vi "Yokogawa - measurement test.vi"() -> ()   [LabVIEW 2013]
uses:
  <instrlib>/Yokogawa PZ4000/Yokogawa PZ4000.lvlib
  electrical2.ctl
panel:
  in  "Module to save":i32=1 min=1 max=4 step=1
  in  "error in (no error)":errorcluster
  out "Electrical Data 3":T1={"Time Stamp"=timestamp(0 s since 1904-01-01), "Temperature (C)"=0.0, "Electrical Data"=[["   NaN", "   NaN", "   NaN", "   NaN"], ["   NaN", "   NaN", "   NaN", "   NaN"], ["   NaN", "   NaN", "   NaN", "   NaN"], ["   NaN", "   NaN", "   NaN", "   NaN"], ["   NaN", "   NaN", "   NaN", "   NaN"], ["   NaN", "   NaN", "   NaN", "   NaN"], ["   NaN", "   NaN", "   NaN", "   NaN"], ["   NaN", "   NaN", "   NaN", "   NaN"], ["   NaN", "   NaN", "   NaN", "   NaN"], ["   NaN", "   NaN", "   NaN", "   NaN"]], "Waveform Graph"=[]}
  in  "Mode (0: Normal)":u16(ring) items=["Normal", "Harmonics"]
  in  "Observation Time":u16(ring)=10 items=["1ksec", "400sec", "200sec", "100sec", "40sec", "20sec", "10sec", "4sec", "2sec", "1sec", "400msec", "200msec", "100msec", "40msec", "20msec", "10msec", "4msec", "2msec", "1msec", "400usec", "200usec", "100usec", "40usec", "20usec", "10usec"]
  in  "Modules on/off":T2
  in  "VISA resource name":refnum<visa-resource-name>
  in  "Current":T3={"A Range (2)"=7, "A Terminal (0: 5A)"=0, "Element (0: ALL)"=0} {"Element (0: ALL)" items=["All", "Element 1", "Element 2", "Element 3", "Element 4"]; "A Terminal (0: 5A)" items=["5A", "20A", "Sensor"]; "A Range (2)" items=["AUTO", "0.1", "0.2", "0.4", "1", "2", "4", "10", "20", "40", "100"]}
  in  "Voltage":T4={"Element (0: All)"=0, "V Range (200)"=4} {"V Range (200)" items=["AUTO", "30", "60", "120", "200", "300", "600", "1200", "2000"]; "Element (0: All)" items=["All", "Element 1", "Element 2", "Element 3", "Element 4"]}
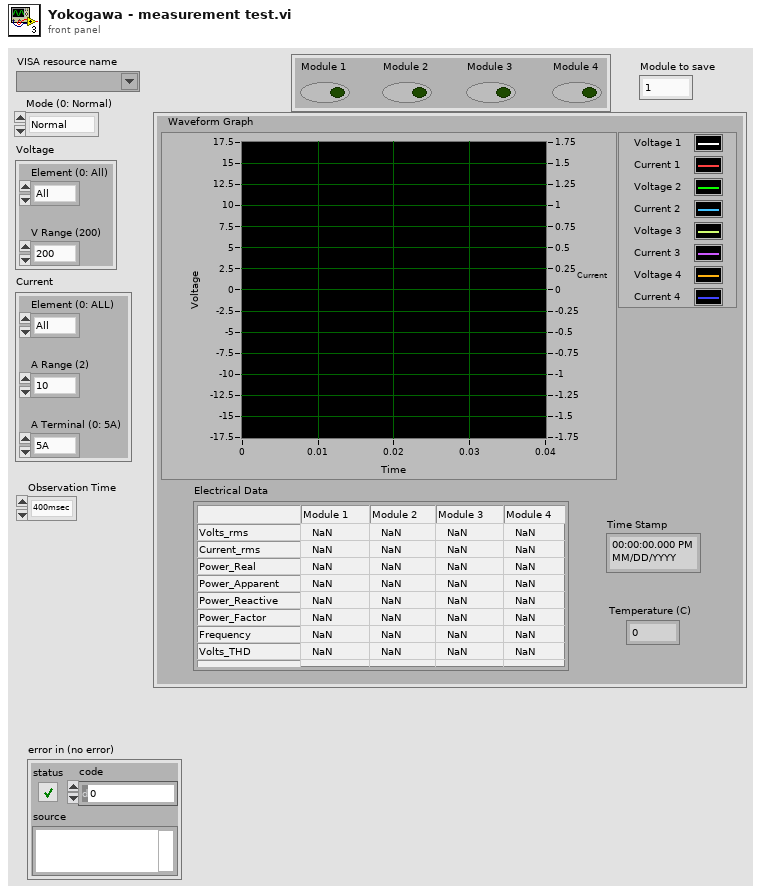
[diagram p1: front panel]
types:
  T1 = typedef "electrical2.ctl" = cluster{"Time Stamp":timestamp, "Temperature (C)":dbl, "Electrical Data":string[][], "Waveform Graph":waveform(dbl)[]}
  T2 = cluster{"Module 1":bool, "Module 2":bool, "Module 3":bool, "Module 4":bool}
  T3 = cluster{"A Range (2)":u16, "A Terminal (0: 5A)":u16, "Element (0: ALL)":u16}
  T4 = cluster{"Element (0: All)":u16, "V Range (200)":u16}
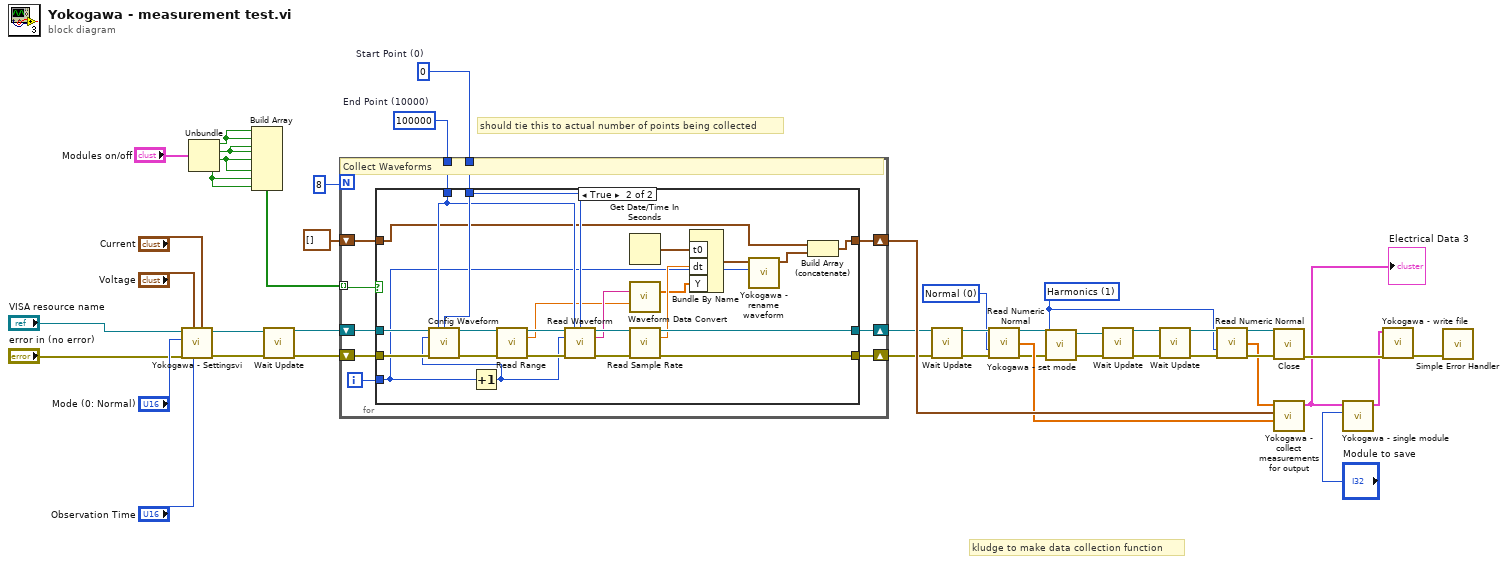
[diagram p0: block diagram]
diagram:
  w38 = u32 100000  # End Point (10000)
  w39 = u32 0  # Start Point (0)
  w8 = u16 1 items=["Normal", "Harmonics"] ("Mode (0: Normal)  2")
  w15 = u16 0 items=["Normal", "Harmonics"] ("Mode (0: Normal)")
  # "should tie this to actual number of points being collected"
  # "kludge to make data collection function"
  n1 = call "Yokogawa - Settingsvi.vi"(5:"Current", 6:"Observation Time", 7:"Voltage", "error in (no error)"="error in (no error)", 10:"Mode (0: Normal)", "Hardware Configuration"="VISA resource name") -> ("error out 2"=w20:errorcluster, "VISA resource name out"=w21:refnum<visa-resource-name>)  [unwired: 4 in]
  n2 = Unbundle("Modules on/off") -> ("Module 1"=w32:bool, "Module 2"=w31:bool, "Module 3"=w30:bool, "Module 4"=w29:bool)
  n3 = Build Array(w32, w32, w31, w31, w30, w30, w29, w29) -> (w34:bool[])
  n4 = call <instrlib>:"Wait Update.vi"("VISA resource name"=w21, "error in (no error)"=w20) -> ("VISA resource name out"=w37:refnum<visa-resource-name>, "error out"=w36:errorcluster)  [unwired: 12 in]
  n5 = for {
    N: 8 -> [_]
    tunnel: w39 -> [w54]
    tunnel: w38 -> [w53]
    shift-right: [w50] -> w24
    shift-left: w37 -> [w52]
    shift-right: [w49] -> w23
    shift-left: w36 -> [w51]
    shift-right: [w47] -> w27
    shift-left: waveform(dbl)[] [] -> [w46]
    tunnel: w34 -> [w45] mode=indexing
    i -> [w48]
    # "Collect Waveforms"
    n6 = case shown="True" w45 {
      tunnel: w54 -> [_ w80]
      tunnel: w53 -> [_ w77]
      tunnel: w52 -> [w56 w75]
      tunnel: w51 -> [w55 w74]
      tunnel: [w56 w70] -> w50
      tunnel: [w55 w69] -> w49
      tunnel: w48 -> [_ w58]
      tunnel: [w57 w67] -> w47
      tunnel: w46 -> [w57 w66]
      frame False {
      }
      frame True {
        n7 = Increment(x=w58) -> (x+1=w59:i32)
        n8 = call <instrlib>:"Config Waveform.vi"("VISA resource name"=w75, "End Point (1000)"=w77, "Start Point (0)"=w80, "Select Trace (1)"=w59, "error in (no error)"=w74) -> ("VISA resource name out"=w73:refnum<visa-resource-name>, "error out"=w78:errorcluster)  [unwired: 9 in]
        n9 = call <instrlib>:"Read Range.vi"("VISA resource name"=w73, "error in (no error)"=w78) -> ("VISA resource name out"=w72:refnum<visa-resource-name>, "Range"=w65:dbl, "error out"=w76:errorcluster)  [unwired: 11 in]
        n10 = call <instrlib>:"Read Waveform.vi"("VISA resource name"=w72, "End Point (1000)"=w77, "Start Point (0)"=w80, "Select Trace (1)"=w59, "error in (no error)"=w76) -> ("VISA resource name out"=w71:refnum<visa-resource-name>, "Waveform Data"=w68:string, "error out"=w79:errorcluster)  [unwired: 8 in]
        n11 = Get Date/Time In Seconds() -> (seconds since 1Jan1904=w62:timestamp)
        n12 = call <instrlib>:"Waveform Data Convert.vi"("Input Data"=w68, "Range"=w65) -> ("Output"=w63:dbl[])  [unwired: 11 in, 2 out]
        n13 = call <instrlib>:"Read Sample Rate.vi"("VISA resource name"=w71, "error in (no error)"=w79) -> ("VISA resource name out"=w70:refnum<visa-resource-name>, "Delta T"=w64:dbl, "error out"=w69:errorcluster)  [unwired: 11 in]
        n14 = Bundle By Name("t0"=w62, "dt"=w64, "Y"=w63) -> (w61:waveform(dbl))  [unwired: 1 in]
        n15 = call "Yokogawa - rename waveform.vi"("Numeric"=w58, "Waveform in"=w61) -> ("Waveform out"=w60:waveform(dbl))  [unwired: 9 in]
        n16 = Build Array (concatenate)(w66, w60) -> (w67:waveform(dbl)[])
      }
    }
  }
  n17 = call <instrlib>:"Wait Update.vi"("VISA resource name"=w24, "error in (no error)"=w23) -> ("VISA resource name out"=w25:refnum<visa-resource-name>, "error out"=w26:errorcluster)  [unwired: 12 in]
  n18 = call <instrlib>:"Read Numeric Normal.vi"("VISA resource name"=w25, "Mode (0: Normal)"=w15, "error in (no error)"=w26) -> ("VISA resource name out"=w19:refnum<visa-resource-name>, "Measure"=w22:dbl[], "error out"=w18:errorcluster)  [unwired: 9 in, 1 out]
  n19 = call "Yokogawa - set mode.vi"("error in (no error)"=w18, "Mode (0: Normal)"=w8, "VISA Refnum in"=w19) -> ("error out"=w9:errorcluster, "VISA Refnum out"=w12:refnum<visa-resource-name>)  [unwired: 7 in]
  n20 = call <instrlib>:"Wait Update.vi"("VISA resource name"=w12, "error in (no error)"=w9) -> ("VISA resource name out"=w11:refnum<visa-resource-name>, "error out"=w10:errorcluster)  [unwired: 12 in]
  n21 = call <instrlib>:"Wait Update.vi"("VISA resource name"=w11, "error in (no error)"=w10) -> ("VISA resource name out"=w14:refnum<visa-resource-name>, "error out"=w13:errorcluster)  [unwired: 12 in]
  n22 = call <instrlib>:"Read Numeric Normal.vi"("VISA resource name"=w14, "Mode (0: Normal)"=w8, "error in (no error)"=w13) -> ("VISA resource name out"=w17:refnum<visa-resource-name>, "Measure"=w7:dbl[], "error out"=w16:errorcluster)  [unwired: 9 in, 1 out]
  n23 = call <instrlib>:"Close.vi"("VISA resource name"=w17, "error in (no error)"=w16) -> ("error out"=w5:errorcluster)  [unwired: 13 in]
  n24 = call "Yokogawa - collect measurements for output.vi"("Normal Measurements"=w22, "Waveforms In"=w27, "Harmonic Measurements"=w7) -> ("Electrical Data Out"=w3:T1)  [unwired: 8 in]
  "Electrical Data 3" <- w3
  n25 = call "Yokogawa - single module.vi"("Module to save"="Module to save", "Electrical Data Out in"=w3) -> ("Electrical Data Out out"=w2:T1)  [unwired: 9 in]
  n26 = call "Yokogawa - write file.vi"("error in (no error)"=w5, "Metadata"=w2) -> ("error out"=w4:errorcluster)  [unwired: 8 in, 1 out]
  n27 = call <vilib>:"Simple Error Handler.vi"("error in (no error)"=w4) -> ()  [unwired: 4 in, 5 out]
